vi "LVClass_ComputePhaseSet GetModalFilter.vi"(0 "ComputePhaseSet in":refnum<class "ComputePhaseSet.lvclass">, 11 "error in (no error)":errorcluster) -> (4 "ComputePhaseSet out":refnum<class "ComputePhaseSet.lvclass">, 6 "polynomial_number_to_filter":u32[](array[numeric]), 15 "error out":errorcluster)   [LabVIEW 2020, in "ComputePhaseSet.lvclass"]
doc: "Get filter for phase reconstruction from Modal decomposition. The filter is\ndefined by the indices of polynomials that must be filtered.\n\n<B>ComputePhaseSetIn</B> : ComputePhaseSet object.\n<B>ComputePhaseSetOut</B> : ComputePhaseSet object.\n<B>nb_coeffs_to_filter</B> : Number of the coefficients to filter in the polynomial base.\n<B>coeffs_to_filter</B> : List of indices of the coefficients to filter in the polynomial base."
uses:
  ComputePhaseSet.lvclass
  ComputePhaseSet.lvclass/ComputePhaseSet.ctl
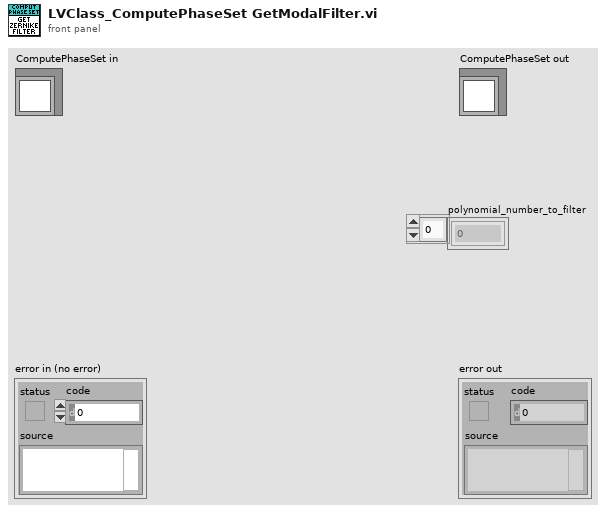
[diagram p1: front panel]
types:
  T1 = typedef "ClassID.ctl" = i64
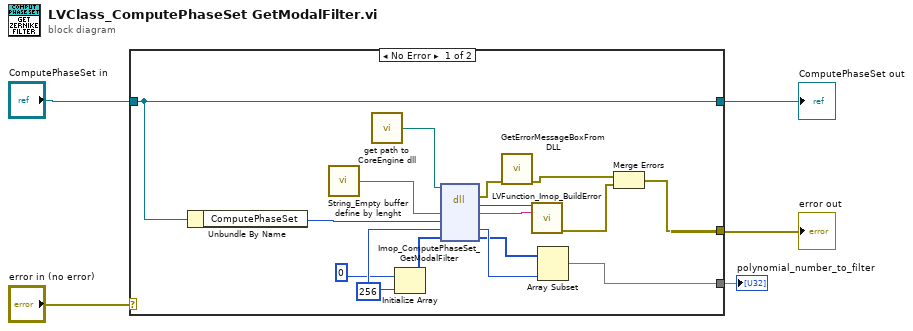
[diagram p0: block diagram]
diagram:
  n1 = case shown="No Error" "error in (no error)" {
    selector: "error in (no error)" -> [_ w23]
    tunnel: [w12 w23] -> w2
    tunnel: [w16 w22] -> w4
    tunnel: "ComputePhaseSet in" -> [w16 w22]
    tunnel: [w6 _] -> w1
    frame No Error {
      w11 = 256
      n2 = Unbundle By Name(w16) -> ("ComputePhaseSet"=w15:T1)
      n3 = call "String_Empty buffer define by lenght.vi"() -> ("Empty buffer"=w19:string)  [unwired: 1 in]
      n4 = call "get path to CoreEngine dll.vi"() -> ("path to wavekit library"=w18:path)  [unwired: 14 in, 1 out]
      n5 = Initialize Array(0, w11) -> (w10:i32[])
      n6 = dll-call lib="D:/2_trunk/Soft_haso/ImOpCoreEngine4_LV2011/DLLs/ImopEngine4_vc100.dll" fn="Imop_ComputePhaseSet_GetModalFilter"(path in=w18, "message"=w19, "objet"=w15, "nb_polynomial"=w11, "polynomial_number_to_filter"=w10) -> (error out=w17:errorcluster, "return type"=w21:i32, "message"=w20:string, "nb_polynomial"=w8:u32, "polynomial_number_to_filter"=w7:u32[])  [unwired: 3 in, 1 out]
      n7 = call "GetErrorMessageBoxFromDLL.vi"("error IN"=w17) -> ("error OUT"=w14:errorcluster)  [unwired: 10 in]
      n8 = call "LVFunction_Imop_BuildError.vi"("code"=w21, "String to Prepend to source (\"\")"=w20) -> ("error out"=w13:errorcluster)  [unwired: 13 in]
      n9 = Array Subset(array=w7, length=w8) -> (w6:u32[])  [unwired: 1 in]
      n10 = Merge Errors(w14, w13) -> (w12:errorcluster)
    }
    frame Error {
    }
  }
  "error out" <- w2
  "ComputePhaseSet out" <- w4
  "polynomial_number_to_filter" <- w1
